vi "Control Multiple Valves.vi"(0 "Session Handle in":T2, 1 "Energize?":bool, 5 "Valves":T1[](array[typedef]) items=["GV1"=21, ""=0], 11 "error in (no error)":errorcluster) -> (4 "Session Handle out":T2, 6 "Valves Out":T1[](array[typedef]) items=["GV1"=21, ""=0], 8 "Success?":bool, 15 "error out":errorcluster)   [LabVIEW 2014]
uses:
  Typedefs/Session Handle.ctl
  PAS.lvclass
  Typedefs/Valves.ctl
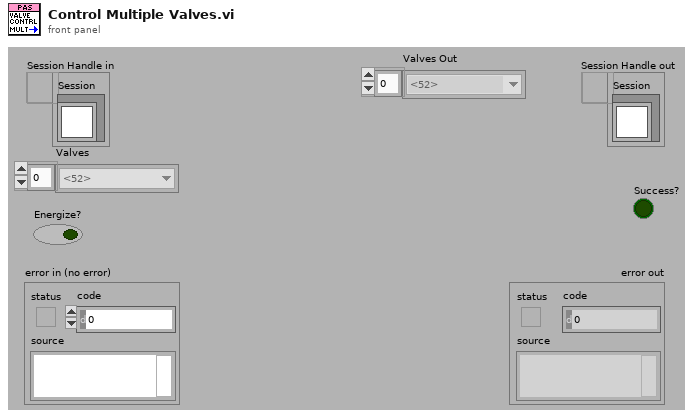
[diagram p1: front panel]
types:
  T1 = typedef "PAS.lvclass/Valves.ctl" = u16
  T2 = typedef "PAS.lvclass/Session Handle.ctl" = refnum<data-value>
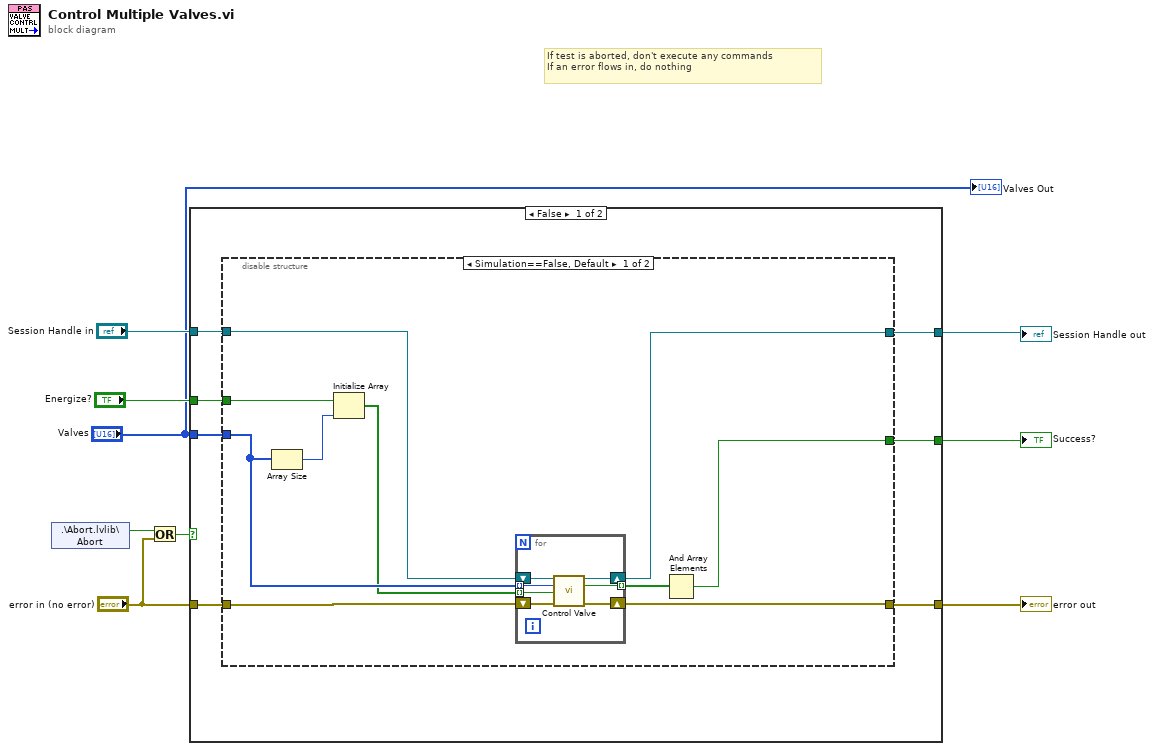
[diagram p0: block diagram]
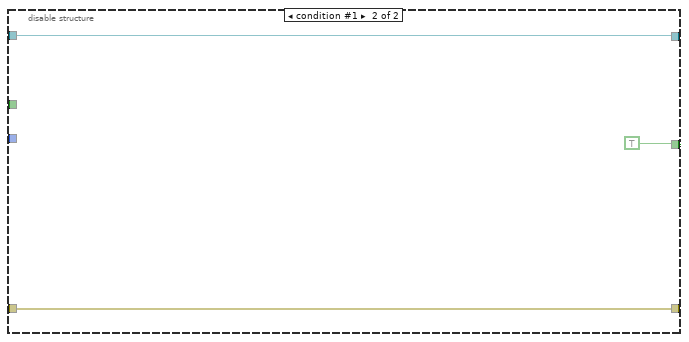
[diagram p2: hidden frame]
diagram:
  # "If test is aborted, don't execute any commands\nIf an error flows in, do nothing"
  n1 = shared-variable ".\\Abort.lvlib\\Abort"() -> (w6:bool)  [unwired: 1 in, 1 out]
  n2 = Or(x=w6, y="error in (no error)") -> (x .or. y?=w4:bool)
  n3 = case shown="False" w4 {
    tunnel: [w16 w38] -> w8
    tunnel: [w15 w37] -> w7
    tunnel: "Session Handle in" -> [w14 w38]
    tunnel: "error in (no error)" -> [w13 w37]
    tunnel: [w12 _] -> w3
    tunnel: "Energize?" -> [w11 _]
    tunnel: "Valves" -> [w10 _]
    frame False {
      n4 = disable-structure shown="Simulation==False, Default" {
        disable-tunnel: [w19 w36] -> w16
        disable-tunnel: [w17 w35] -> w15
        disable-tunnel: w14 -> [w23 w36]
        disable-tunnel: w13 -> [w24 w35]
        disable-tunnel: [w18 TRUE] -> w12
        disable-tunnel: w11 -> [w26 _]
        disable-tunnel: w10 -> [w22 _]
        frame condition #0 (active) {
          n5 = Array Size(array=w22) -> (size(s)=w25:i32)
          n6 = Initialize Array(w26, w25) -> (w21:bool[])
          n7 = for {
            shift-right: [w31] -> w19
            shift-left: w23 -> [w32]
            shift-right: [w30] -> w17
            shift-left: w24 -> [w33]
            tunnel: w22 -> [w29] mode=indexing
            tunnel: w21 -> [w28] mode=indexing
            tunnel: [w27] -> w20 mode=indexing
            n8 = call "Control Valve.vi"("Session Handle in"=w32, "Valves"=w29, "Energize?"=w28, "error in (no error)"=w33) -> ("Session Handle out"=w31:T2, "Success?"=w27:bool, "error out"=w30:errorcluster)  [unwired: 8 in, 1 out]
          }
          n9 = And Array Elements(Boolean array=w20) -> (logical AND=w18:bool)
        }
        frame condition #1 {
        }
      }
    }
    frame True {
    }
  }
  "Session Handle out" <- w8
  "error out" <- w7
  "Success?" <- w3
  "Valves Out" <- "Valves"
